vi "SVN Version.vi"(8 "error in (no error)":errorcluster) -> (0 "error out":errorcluster, 1 "Version string":string, 2 "Revision":i32, 3 "standard output":string, 4 "Successful Version Check":bool)   [LabVIEW 2015]
uses:
  <vilib>/Utility/config.llb/NI_LVConfig.lvlib
  <vilib>/Utility/config.llb/Read Key (Boolean).vi
panel:
  in  "initial string":string="The version number of the MathCAD files used to create this design is"
  in  "Repository URL":string="https://forge.cornell.edu/svn/repos/automated_design/Final Designs/"
  in  "command":string="cmd /c svn info"
  in  "working directory":path=path "C:/Program Files/CollabNet Subversion Client"
  # "cmd /c svn status  --show-updates wc"
  # "$ svn checkout -r 2 file:///var/svn/repos/test mine"
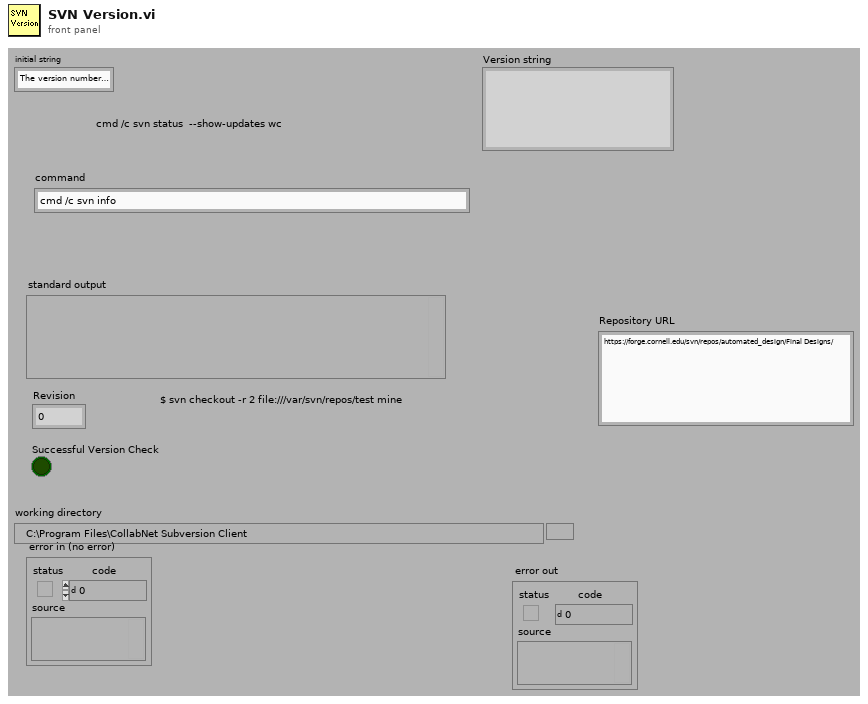
[diagram p1: front panel]
types:
  T1 = typedef "NI_LVConfig.lvlib/Config Data RefNum.ctl" = refnum<k1>
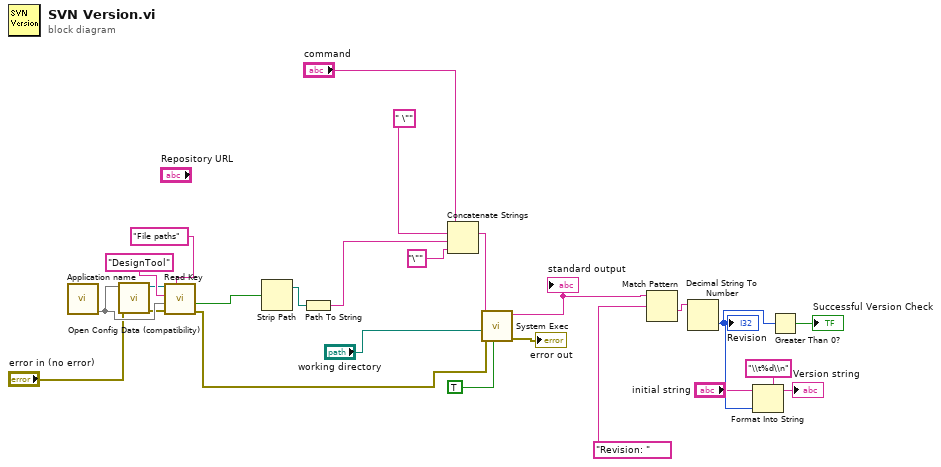
[diagram p0: block diagram]
diagram:
  n1 = call "Application name.vi"() -> (0:w20)  [unwired: 4 in, 3 out]
  n2 = call <vilib>:"Open Config Data (compatibility).vi"("error in (no error)"="error in (no error)", "configuration file path"=w20) -> ("error out"=w9:errorcluster, "refnum"=w22:T1)  [unwired: 7 in, 1 out]
  n3 = call-poly <vilib>:"Read Key.vi"("section"="File paths", "error in (no error)"=w9, "default value"=w20, "key"="DesignTool", "refnum"=w22) -> ("error out"=w7:errorcluster, "value"=w10:bool)  [unwired: 3 in, 2 out]
  n4 = Strip Path(path=w10) -> (stripped path=w19:path)  [unwired: 1 out]
  n5 = Path To String(path=w19) -> (string=w18:string)
  n6 = Concatenate Strings("command", " \"" ("string"), w18, "\"" ("string")) -> (w5:string)
  n7 = call <vilib>:"System Exec.vi"("run minimized? (F)"=TRUE, "error in (no error)"=w7, "working directory"="working directory", "command line"=w5) -> ("error out"=→"error out":errorcluster, "standard output"=w15:string)  [unwired: 4 in, 2 out]
  "standard output" <- w15
  n8 = Match Pattern(string=w15, regular expression="Revision: ") -> (after substring=w13:string)  [unwired: 1 in, 3 out]
  n9 = Decimal String To Number(string=w13) -> (number=w3:i32)  [unwired: 2 in, 1 out]
  "Revision" <- w3
  n10 = Format Into String(format string="\\t%d\\n", initial string="initial string", w3) -> (resulting string=→"Version string":string)  [unwired: 1 in, 1 out]
  n11 = Greater Than 0?(x=w3) -> (x > 0?=→"Successful Version Check":bool)
